vi "Send Configure AC Bandwidth [AC].vi"(7 "Message Priority (Normal)":T1=enum."Normal", 8 "error in (no error)":errorcluster, 9 "ac max frequency (300.0E+3 Hz)":dbl=300000.0 format="%^.2e", 10 "ac min frequency (20.0 Hz)":dbl=20.0 format="%^.2e", 11 "Message Enqueuer":refnum<class "Message Enqueuer.lvclass">) -> (0 "error out":errorcluster, 3 "Message Enqueuer out":refnum<class "Message Enqueuer.lvclass">)   [LabVIEW 2015, in "CS++DMM.lvlib" / "Configure AC Bandwidth [AC] Msg.lvclass"]
doc: "Sends the <B>CS++DMM.lvlib:Configure AC Bandwidth [AC] Msg.lvclass</B> message.\n\n<B>CS++DMM.lvlib:CS++DMM.lvclass:Configure AC Bandwidth [AC].vi</B> Description:\n\nThis VI configures the AC minimum and maximum frequency for DMMs that take AC voltage or AC current measurements.\n\nThis VI affects the behavior of the instrument only if the IviDmm>Basic Operation>Function property is set to an AC voltage or AC current measurement.\n\nNote:\n\n(1) This VI is part of the IviDmmACMeasurement [AC] extension group."
uses:
  Configure AC Bandwidth [AC] Msg.lvclass
  <vilib>/ActorFramework/Message Enqueuer/Message Enqueuer.lvclass
  <vilib>/ActorFramework/Message Enqueuer/Message Priority.ctl
  Configure AC Bandwidth [AC] Msg.lvclass/Configure AC Bandwidth [AC] Msg.ctl
  <vilib>/ActorFramework/Message Enqueuer/Message Enqueuer.lvclass/Message Enqueuer.ctl
  <vilib>/ActorFramework/Message Priority Queue/Priority Enqueue.vi
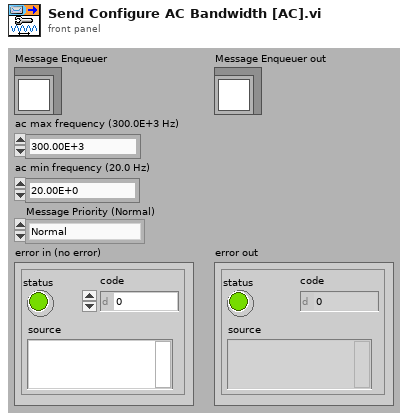
[diagram p1: front panel]
types:
  T1 = typedef "Actor Framework.lvlib/Message Enqueuer.lvclass/Message Priority.ctl" = enum16{"Low", "Normal", "High"}
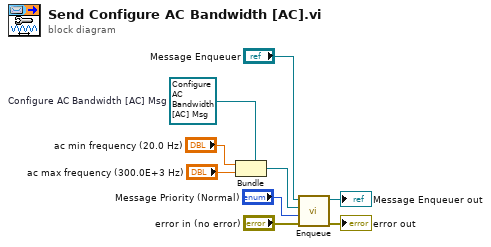
[diagram p0: block diagram]
diagram:
  w3 = refnum<class "Configure AC Bandwidth [AC] Msg.lvclass"> refnum  # Configure AC Bandwidth [AC] Msg
  n1 = Bundle(cluster=w3, "ac min frequency (20.0 Hz)", "ac max frequency (300.0E+3 Hz)") -> (w6:refnum<class "Configure AC Bandwidth [AC] Msg.lvclass">)
  n2 = call <vilib>:"Enqueue.vi"("error in (no error)"="error in (no error)", "Message Priority (Normal)"="Message Priority (Normal)", "Message"=w6, "Message Enqueuer in"="Message Enqueuer") -> ("error out"=→"error out":errorcluster, "Message Enqueuer out"=→"Message Enqueuer out":refnum<class "Message Enqueuer.lvclass">)  [unwired: 6 in]
